vi "BT DUT Update Payload Length.vi"(8 "error in (no error)":errorcluster, 11 "niDTS BT DUT in":refnum<class "niDTS BT Dut.lvclass">) -> (0 "error out":errorcluster, 3 "niDTS BT DUT out":refnum<class "niDTS BT Dut.lvclass">)   [LabVIEW 2015, in "niDTS BT.lvlib" / "niDTS BT Dut.lvclass"]
doc: "Updates the payload length to comply with DUT settings. If 16 symbols is set to TRUE, this sets the payload length according to the Standard, Rate, Streams, and Bandwidth. If 16 symbols is FALSE, the payload length is not modified. In both cases, the actual payload length is coerced by Payload Length Limit if required."
uses:
  niDTS BT Dut.lvclass
  niDTS BT Dut.lvclass/niDTS BT Dut.ctl
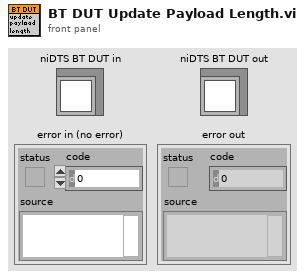
[diagram p1: front panel]
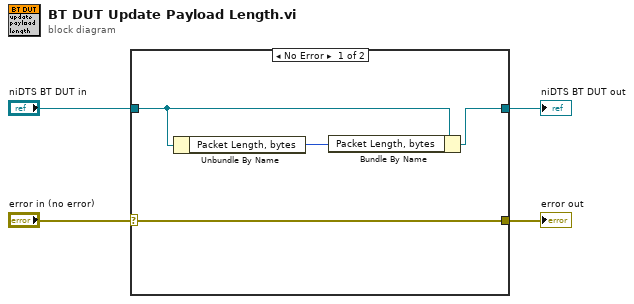
[diagram p0: block diagram]
diagram:
  n1 = case shown="No Error" "error in (no error)" {
    selector: "error in (no error)" -> [w8 w10]
    tunnel: [w8 w10] -> w3
    tunnel: [w6 w9] -> w1
    tunnel: "niDTS BT DUT in" -> [w5 w9]
    frame No Error {
      n2 = Unbundle By Name(w5) -> ("Packet Length, bytes"=w7:i32)
      n3 = Bundle By Name(cluster=w5, "Packet Length, bytes"=w7) -> (w6:refnum<class "niDTS BT Dut.lvclass">)
    }
    frame Error {
    }
  }
  "error out" <- w3
  "niDTS BT DUT out" <- w1
